vi "Robot Systems.vi"(11 "output cluster":T1) -> ()   [LabVIEW 2016]
uses:
  Joystick/ControlsToCommands.ctl
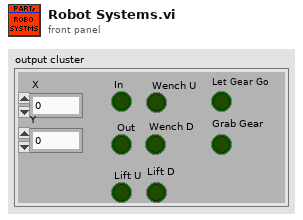
[diagram p1: front panel]
types:
  T1 = typedef "ControlsToCommands.ctl" = cluster{"X":dbl, "Y":dbl, "In":bool, " Out":bool, "Lift U":bool, " Wench U":bool, " Wench D":bool, "Lift D":bool, "Let Gear Go":bool, "Grab Gear":bool}
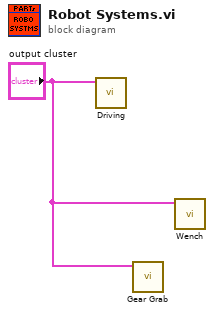
[diagram p0: block diagram]
diagram:
  n1 = call "Driving.vi"("output cluster"="output cluster") -> ()  [unwired: 11 in]
  n2 = call "Gear Grab.vi"("output cluster"="output cluster") -> ()  [unwired: 11 in]
  n3 = call "Wench.vi"("output cluster"="output cluster") -> ()  [unwired: 11 in]
